vi "temperatur.vi"(8 "error in":errorcluster, 11 "Start":bool) -> (0 "error out":errorcluster, 2 "done":bool, 3 "Temperatur":dbl)   [LabVIEW 2013, in "TempHygro.lvlib"]
uses:
  lib/TempHygro.lvlib
  <vilib>/DAQmx/create/channels.llb/DAQmx Create Channel (AI-Voltage-Basic).vi
  <vilib>/DAQmx/read.llb/DAQmx Read (Analog DBL 1Chan 1Samp).vi
panel:
  in  "U_gesamt":dbl=8.0 format="%#_13g"
  out "Numeric":dbl format="%#_13g"
  out "Ug - U_NTC":dbl
  out "widerstand":dbl
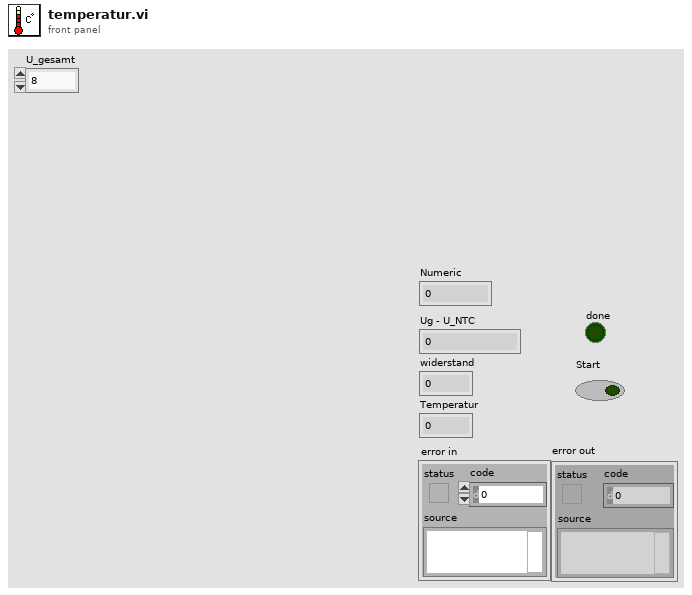
[diagram p1: front panel]
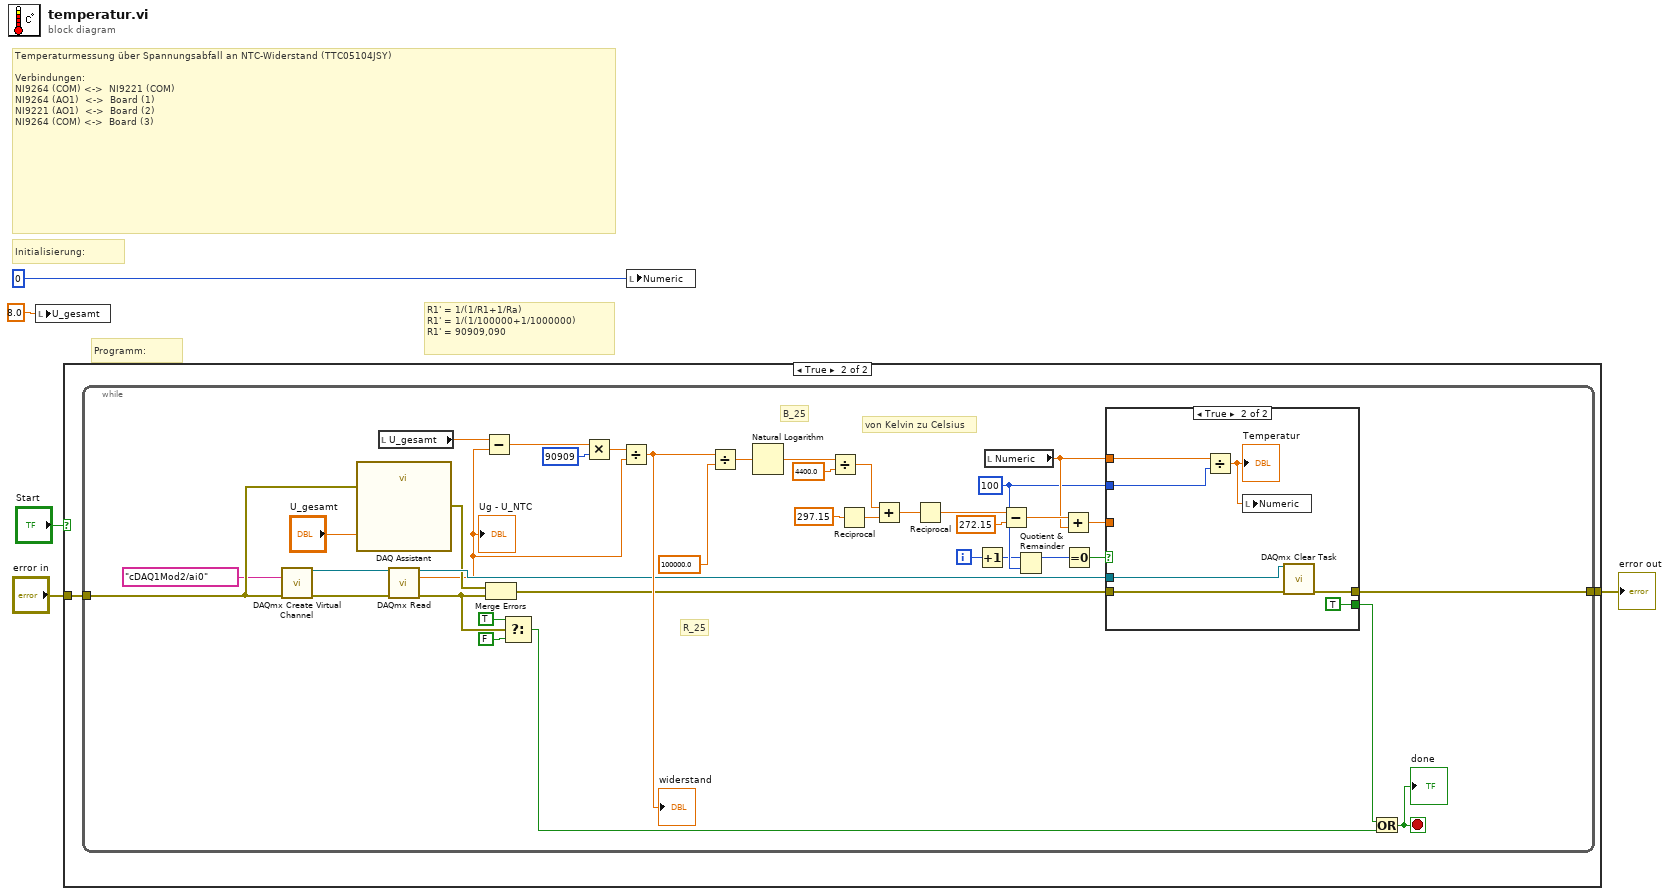
[diagram p0: block diagram]
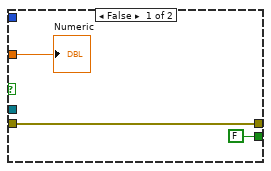
[diagram p3: hidden frame]
diagram:
  # "R1' = 1/(1/R1+1/Ra) \nR1' = 1/(1/100000+1/1000000) \nR1' = 90909,090"
  # "Programm:"
  # "Initialisierung:"
  # "Temperaturmessung über Spannungsabfall an NTC-Widerstand (TTC05104JSY)\n\nVerbindungen:  \nNI9264 (COM) <->  NI9221 (COM)\nNI9264 (AO1)  <->  Board (1)\nNI9221 (AO1)  <->  Board (2)\nNI9264 (COM) <->  Board (3)"
  n1 = local write "U_gesamt"(8.0 ("U_gesamt")) -> ()
  n2 = case shown="True" "Start" {
    tunnel: "error in" -> [w6 w8]
    tunnel: [w6 w7] -> w1
    frame False {
    }
    frame True {
      n3 = while {
        tunnel: w8 -> [w22]
        tunnel: [w19] -> w7
        i -> [w26]
        stop <- w13 stop-if-true
        w29 = 100 ("y")
        # "von Kelvin zu Celsius"
        # "B_25"
        # "R_25"
        n4 = call-poly <vilib>:"DAQmx Create Virtual Channel.vi"("physical channels"=tag "cDAQ1Mod2/ai0", "error in"=w22) -> ("task out"=w28:refnum<k21>, "error out"=w21:errorcluster)  [unwired: 12 in]
        n5 = call "DAQ Assistant"("data"="U_gesamt", "error in"=w22) -> ("error out"=w20:errorcluster)  [unwired: 16 in, 1 out]
        n6 = local read "U_gesamt"() -> (w27:dbl)
        n7 = call-poly <vilib>:"DAQmx Read.vi"("task/channels in"=w28, "error in"=w21) -> ("task out"=w23:refnum<k21>, "data"=w9:dbl, "error out"=w16:errorcluster)  [unwired: 11 in]
        "Ug - U_NTC" <- w9
        n8 = Subtract(x=w27, y=w9) -> (x-y=w10:dbl)
        n9 = Merge Errors(w20, w16) -> (w18:errorcluster)
        n10 = Select(t=TRUE, s=w16, f=FALSE) -> (s? t:f=w12:bool)
        n11 = Multiply(x=w10, y=90909) -> (x*y=w46:dbl)
        n12 = Divide(x=w46, y=w9) -> (x/y=w37:dbl)
        "widerstand" <- w37
        n13 = Divide(x=w37, y=100000.0) -> (x/y=w44:dbl)
        n14 = Natural Logarithm(1:w44) -> (0:w43:dbl)
        n15 = Divide(x=w43, y=4400.0) -> (x/y=w41:dbl)
        n16 = Reciprocal(x=297.15 ("y")) -> (1/x=w38:dbl)
        n17 = Add(x=w41, y=w38) -> (x+y=w40:dbl)
        n18 = Reciprocal(x=w40) -> (1/x=w36:dbl)
        n19 = Increment(x=w26) -> (x+1=w25:i32)
        n20 = local read "Numeric"() -> (w33:dbl)
        n21 = Subtract(x=w36, y=272.15) -> (x-y=w34:dbl)
        n22 = Quotient & Remainder(x=w25, y=w29) -> (x-y*floor(x/y)=w32:i32)  [unwired: 1 out]
        n23 = Add(x=w34, y=w33) -> (x+y=w30:dbl)
        n24 = Equal To 0?(x=w32) -> (x = 0?=w31:bool)
        n25 = case shown="True" w31 {
          tunnel: w29 -> [_ w57]
          tunnel: w33 -> [_ w56]
          tunnel: w30 -> [w50 _]
          tunnel: [FALSE TRUE] -> w14
          tunnel: w23 -> [_ w53]
          tunnel: [w48 w52] -> w19
          tunnel: w18 -> [w48 w51]
          frame False {
            "Numeric" <- w50
          }
          frame True {
            n26 = Divide(x=w56, y=w57) -> (x/y=w55:dbl)
            "Temperatur" <- w55
            n27 = local write "Numeric"(w55) -> ()
            n28 = call <vilib>:"DAQmx Clear Task.vi"("task in"=w53, "error in"=w51) -> ("error out"=w52:errorcluster)  [unwired: 13 in]
          }
        }
        n29 = Or(x=w14, y=w12) -> (x .or. y?=w13:bool)
        "done" <- w13
      }
    }
  }
  "error out" <- w1
  n30 = local write "Numeric"(0) -> ()
